vi "4155C Thermopower Transfer Config SMUs.vi"(0 "VISA resource name in":refnum<visa-resource-name>, 1 "sweep method":u16(ring) items=["Continuous", "Pulsed"], 2 "Gate mode":u16(ring) items=["Auto", "Limited", "Fixed"], 3 "Gate Range":u8(slide)=6 max=11 scale=0.0..11.0, 5 "Pulse period":dbl=0.005 min=0.005 max=1.0 step=0.0001 format="%.4f", 7 "Pulse width":dbl=0.0005 min=0.0005 max=0.1 step=0.0001 format="%.4f", 8 "Drain Standby":bool, 9 "Base voltage":dbl format="%^.4e", 10 "Gate Standby":bool, 11 "error in (no error)":errorcluster, 12 "SMU4":cluster{"on/off":bool, "Voltage":dbl} {"Voltage" min=-100.0 max=100.0 format="%.2f"}, 13 "Source/drain mode":u16(ring) items=["Auto", "Limited", "Fixed"], 14 "Source/drain Range":u8(slide)=6 max=11 scale=0.0..11.0) -> (4 "VISA Resource Name out":refnum<visa-resource-name>, 15 "error out":errorcluster)   [LabVIEW 2016]
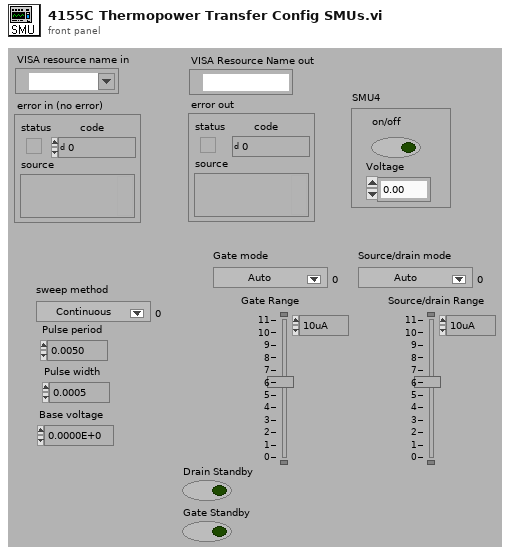
[diagram p1: front panel]
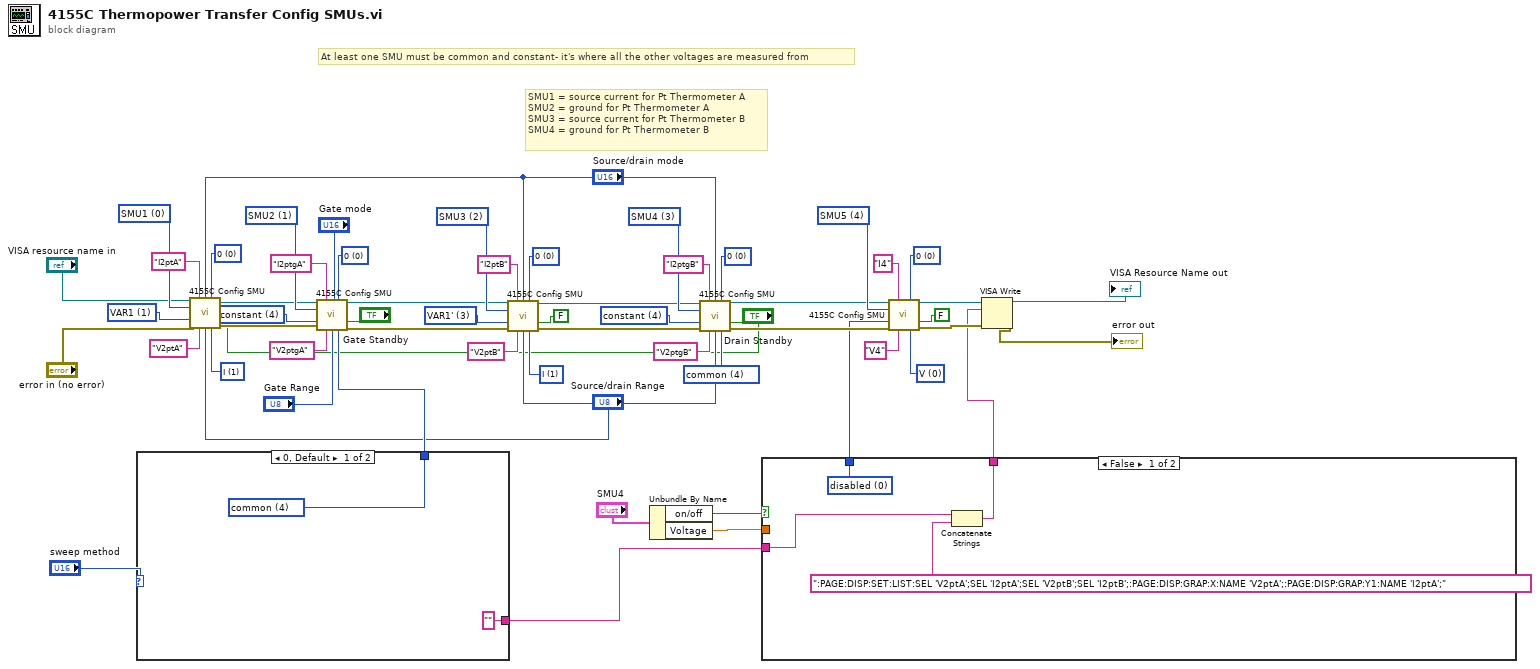
[diagram p0: block diagram]
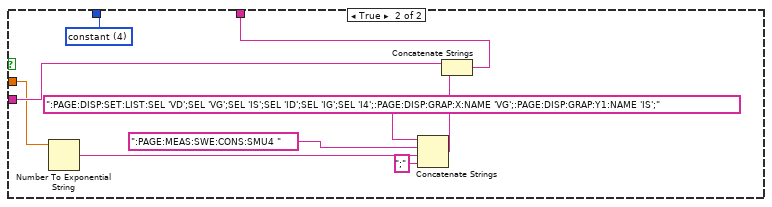
[diagram p2: hidden frame]
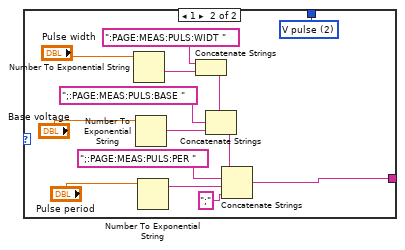
[diagram p3: hidden frame]
diagram:
  w15 = u32 0 items=["SMU1  ", "SMU2  ", "SMU3  ", "SMU4  ", "SMU5  ", "SMU6  "] ("unit to configure")
  w16 = u32 1 items=["disabled  ", "VAR1  ", "VAR2  ", "VAR1'  ", "constant  "] ("function")
  w18 = u32 0 items=["0  ", "10K Ohms  ", "100K Ohms  ", "1M Ohms  "] ("series resistance *")
  w19 = u32 1 items=["V  ", "I  ", "V pulse  ", "I pulse  ", "  common  "] ("mode")
  w37 = u32 0 items=["V  ", "I  ", "V pulse  ", "I pulse  ", "  common  "] ("mode")
  w38 = u32 0 items=["0  ", "10K Ohms  ", "100K Ohms  ", "1M Ohms  "] ("series resistance *")
  w40 = u32 4 items=["SMU1  ", "SMU2  ", "SMU3  ", "SMU4  ", "SMU5  ", "SMU6  "] ("unit to configure")
  w43 = u32 0 items=["0  ", "10K Ohms  ", "100K Ohms  ", "1M Ohms  "] ("series resistance *")
  w10 = u32 4 items=["disabled  ", "VAR1  ", "VAR2  ", "VAR1'  ", "constant  "] ("function")
  w45 = u32 1 items=["SMU1  ", "SMU2  ", "SMU3  ", "SMU4  ", "SMU5  ", "SMU6  "] ("unit to configure")
  w47 = u32 4 items=["V  ", "I  ", "V pulse  ", "I pulse  ", "  common  "] ("mode")
  w48 = u32 0 items=["0  ", "10K Ohms  ", "100K Ohms  ", "1M Ohms  "] ("series resistance *")
  w50 = u32 4 items=["disabled  ", "VAR1  ", "VAR2  ", "VAR1'  ", "constant  "] ("function")
  w51 = u32 3 items=["SMU1  ", "SMU2  ", "SMU3  ", "SMU4  ", "SMU5  ", "SMU6  "] ("unit to configure")
  w54 = u32 1 items=["V  ", "I  ", "V pulse  ", "I pulse  ", "  common  "] ("mode")
  w55 = u32 0 items=["0  ", "10K Ohms  ", "100K Ohms  ", "1M Ohms  "] ("series resistance *")
  w57 = u32 3 items=["disabled  ", "VAR1  ", "VAR2  ", "VAR1'  ", "constant  "] ("function")
  w58 = u32 2 items=["SMU1  ", "SMU2  ", "SMU3  ", "SMU4  ", "SMU5  ", "SMU6  "] ("unit to configure")
  # "SMU1 = source current for Pt Thermometer A\nSMU2 = ground for Pt Thermometer A\nSMU3 = source current for Pt Thermometer B\nSMU4 = ground for Pt Thermometer B"
  # "At least one SMU must be common and constant- it's where all the other voltages are measured from"
  n1 = case shown="0, Default" "sweep method" {
    tunnel: [w60 w74] -> w27
    tunnel: ["" w62] -> w7
    frame 0, Default {
      w60 = u32 4 items=["V  ", "I  ", "V pulse  ", "I pulse  ", "  common  "] ("mode")
    }
    frame 1 {
      w74 = u32 2 items=["V  ", "I  ", "V pulse  ", "I pulse  ", "  common  "] ("mode")
      n2 = Number To Exponential String(number="Pulse width") -> (E-format string=w70:string)  [unwired: 3 out]
      n3 = Number To Exponential String(number="Base voltage") -> (E-format string=w66:string)  [unwired: 3 out]
      n4 = Number To Exponential String(number="Pulse period") -> (E-format string=w63:string)  [unwired: 3 out]
      n5 = Concatenate Strings(":PAGE:MEAS:PULS:WIDT " ("Substring"), w70) -> (w68:string)
      n6 = Concatenate Strings(w68, ";:PAGE:MEAS:PULS:BASE " ("Substring"), w66) -> (w64:string)
      n7 = Concatenate Strings(w64, ";:PAGE:MEAS:PULS:PER " ("Substring"), w63, ";" ("Substring")) -> (w62:string)
    }
  }
  n8 = call "4155C Config SMU.vi"("VISA session"="VISA resource name in", "I name (max 6 chars)"="I2ptA", "Range mode"="Source/drain mode", "series resistance *"=w18, "unit to configure"=w15, "function"=w16, "standby"="Drain Standby", "error in (no error)"="error in (no error)", "V name (max 6 chars)"="V2ptA", "Range"="Source/drain Range", "mode"=w19) -> ("dup VISA resource name"=w13:refnum<visa-resource-name>, "error out"=w14:errorcluster)  [unwired: 3 out]
  n9 = call "4155C Config SMU.vi"("VISA session"=w13, "I name (max 6 chars)"="I2ptgA", "Range mode"="Gate mode", "series resistance *"=w43, "unit to configure"=w45, "function"=w10, "standby"="Gate Standby", "error in (no error)"=w14, "V name (max 6 chars)"="V2ptgA", "Range"="Gate Range", "mode"=w27) -> ("dup VISA resource name"=w24:refnum<visa-resource-name>, "error out"=w23:errorcluster)  [unwired: 3 out]
  n10 = call "4155C Config SMU.vi"("VISA session"=w24, "I name (max 6 chars)"="I2ptB", "Range mode"="Source/drain mode", "series resistance *"=w55, "unit to configure"=w58, "function"=w57, "standby"=FALSE, "error in (no error)"=w23, "V name (max 6 chars)"="V2ptB", "Range"="Source/drain Range", "mode"=w54) -> ("dup VISA resource name"=w34:refnum<visa-resource-name>, "error out"=w33:errorcluster)  [unwired: 3 out]
  n11 = Unbundle By Name("SMU4") -> ("on/off"=w5:bool, "Voltage"=w6:dbl)
  n12 = call "4155C Config SMU.vi"("VISA session"=w34, "I name (max 6 chars)"="I2ptgB", "Range mode"="Source/drain mode", "series resistance *"=w48, "unit to configure"=w51, "function"=w50, "standby"="Drain Standby", "error in (no error)"=w33, "V name (max 6 chars)"="V2ptgB", "Range"="Source/drain Range", "mode"=w47) -> ("dup VISA resource name"=w21:refnum<visa-resource-name>, "error out"=w22:errorcluster)  [unwired: 3 out]
  n13 = case shown="False" w5 {
    tunnel: w7 -> [w77 w87]
    tunnel: [w76 w86] -> w3
    tunnel: w6 -> [_ w84]
    tunnel: [w75 w85] -> w2
    frame False {
      w75 = u32 0 items=["disabled  ", "VAR1  ", "VAR2  ", "VAR1'  ", "constant  "] ("function")
      n14 = Concatenate Strings(w77, ":PAGE:DISP:SET:LIST:SEL 'V2ptA';SEL 'I2ptA';SEL 'V2ptB';SEL 'I2ptB';:PAGE:DISP:GRAP:X:NAME 'V2ptA';:PAGE:DISP:GRAP:Y1:NAME 'I2ptA';" ("write buffer (\"\")")) -> (w76:string)
    }
    frame True {
      w85 = u32 4 items=["disabled  ", "VAR1  ", "VAR2  ", "VAR1'  ", "constant  "] ("function")
      n15 = Number To Exponential String(number=w84) -> (E-format string=w82:string)  [unwired: 3 out]
      n16 = Concatenate Strings(":PAGE:DISP:SET:LIST:SEL 'VD';SEL 'VG';SEL 'IS';SEL 'ID';SEL 'IG';SEL 'I4';:PAGE:DISP:GRAP:X:NAME 'VG';:PAGE:DISP:GRAP:Y1:NAME 'IS';" ("write buffer (\"\")"), ":PAGE:MEAS:SWE:CONS:SMU4 " ("write buffer (\"\")"), w82, ";" ("Substring")) -> (w80:string)
      n17 = Concatenate Strings(w87, w80) -> (w86:string)
    }
  }
  n18 = call "4155C Config SMU.vi"("VISA session"=w21, "I name (max 6 chars)"="I4", "series resistance *"=w38, "unit to configure"=w40, "function"=w2, "standby"=FALSE, "error in (no error)"=w22, "V name (max 6 chars)"="V4", "mode"=w37) -> ("dup VISA resource name"=w32:refnum<visa-resource-name>, "error out"=w31:errorcluster)  [unwired: 2 in, 3 out]
  n19 = VISA Write(VISA resource name=w32, write buffer=w3, error in (no error)=w31) -> (VISA resource name out=→"VISA Resource Name out":refnum<visa-resource-name>, error out=→"error out":errorcluster)  [unwired: 1 out]
